vi "Table-Sort by numerical strings order.vi"(8 "error in (no error)":errorcluster, 9 "Sort By in":enum16{"row", "column"}(ring)=enum."column", 10 "Order (ascending)":enum16{"ascending", "descending"}(ring), 11 "Numerical strings table in":string[][](array[string])=[["55", "111", ""], ["3", "23", ""], ["1", "45", "123"], ["", "", ""], ["", "", ""], ["34", "", ""], ["", "", ""], ["", "", ""]]) -> (0 "error out":errorcluster, 3 "Sorted numerical strings table":string[][](array[string]))   [LabVIEW 2020]
uses:
  <userlib>/_OpenG.lib/array/array.llb/Search 1D Array (String)__ogtk.vi
  <userlib>/_OpenG.lib/array/array.llb/Delete Elements from 1D Array (String)__ogtk.vi
  <userlib>/_OpenG.lib/array/array.llb/Sort 1D Array (I32)__ogtk.vi
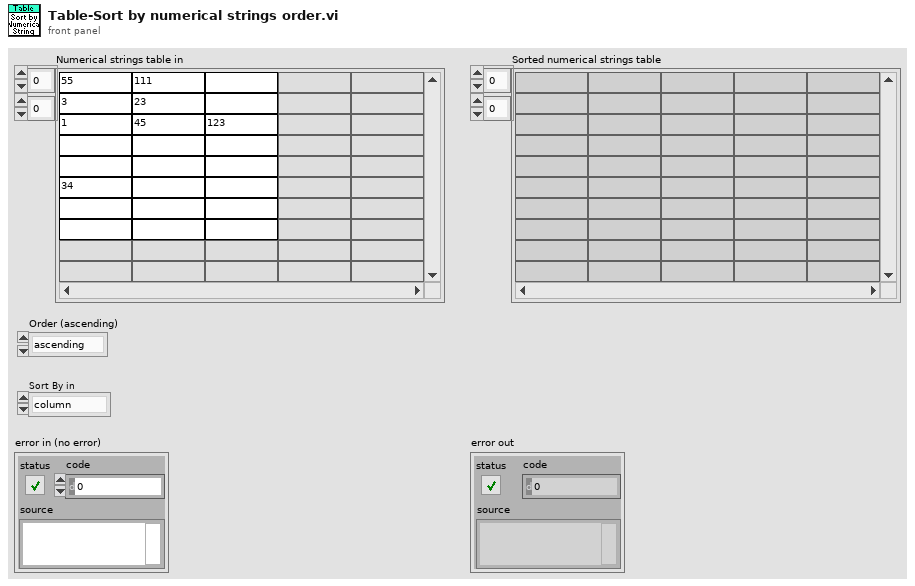
[diagram p1: front panel]
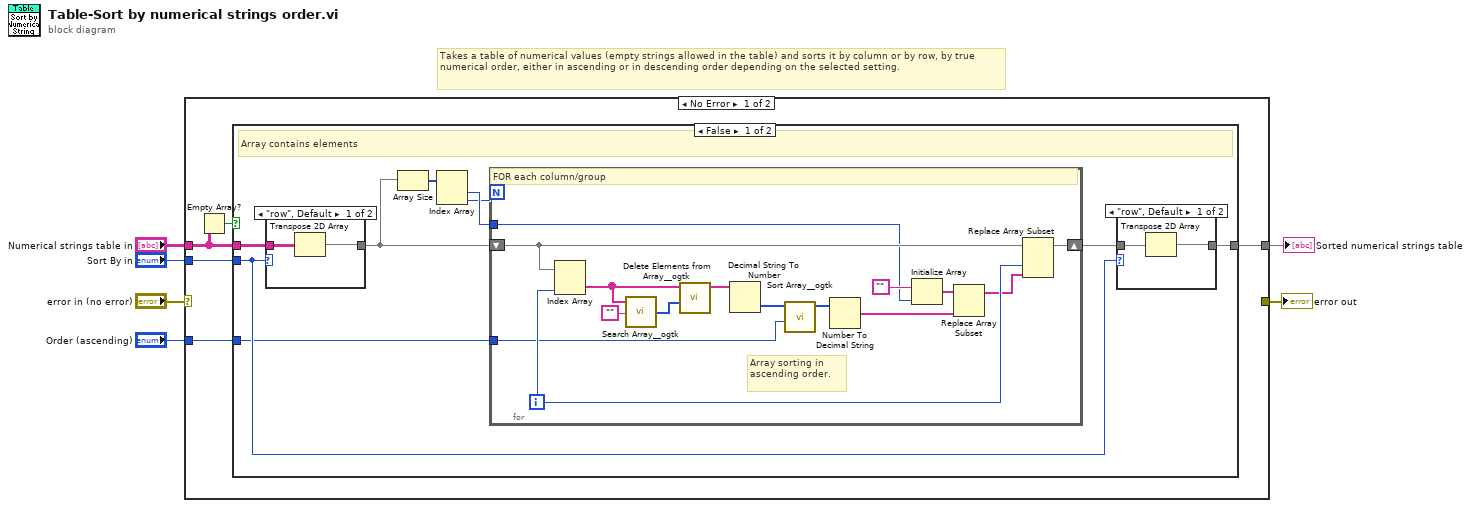
[diagram p0: block diagram]
diagram:
  # "Takes a table of numerical values (empty strings allowed in the table) and sorts it by column or by row, by true numerical order, either in ascending or in descending order depending on the selected setting."
  n1 = case shown="No Error" "error in (no error)" {
    selector: "error in (no error)" -> [_ w42]
    tunnel: [w11 _] -> w6
    tunnel: "Sort By in" -> [w10 _]
    tunnel: "Numerical strings table in" -> [w7 _]
    tunnel: "Order (ascending)" -> [w9 _]
    tunnel: [_ w42] -> w1
    frame No Error {
      n2 = Empty Array?(array=w7) -> (empty?=w8:bool)
      n3 = case shown="False" w8 {
        tunnel: [w15 _] -> w11
        tunnel: w10 -> [w14 _]
        tunnel: w7 -> [w13 _]
        tunnel: w9 -> [w12 _]
        frame False {
          # "Array contains elements"
          n4 = case shown="\"row\", Default" w14 {
            tunnel: w13 -> [w25 w26]
            tunnel: [w24 w26] -> w17
            frame "row", Default {
              n5 = Transpose 2D Array(2D array=w25) -> (transposed array=w24:string[][])
            }
            frame "column" {
            }
          }
          n6 = Array Size(array=w17) -> (size(s)=w20:i32[])
          n7 = Index Array(array=w20) -> (element #1=w19:i32, element #2=w18:i32)  [unwired: 2 in]
          n8 = for {
            N: w18 -> [_]
            shift-right: [w35] -> w16
            shift-left: w17 -> [w33]
            tunnel: w19 -> [w28]
            tunnel: w12 -> [w27]
            i -> [w34]
            # "Array sorting in ascending order."
            # "FOR each column/group"
            n9 = Index Array(array=w33, index (col)=w34) -> (element=w39:string[])  [unwired: 1 in]
            n10 = call-poly <userlib>:"Search Array__ogtk.vi"("Array"=w39, "Element Data"="") -> ("Indices of Elements"=w41:i32[])  [unwired: 7 in]
            n11 = call-poly <userlib>:"Delete Elements from Array__ogtk.vi"("indices"=w41, "array"=w39) -> ("array w/ subset deleted"=w38:string[])  [unwired: 8 in, 1 out]
            n12 = Decimal String To Number(string=w38) -> (number=w37:i32[])  [unwired: 2 in, 1 out]
            n13 = call-poly <userlib>:"Sort Array__ogtk.vi"("Order"=w27, "Array in"=w37) -> ("Sorted Array out"=w36:i32[])  [unwired: 8 in, 1 out]
            n14 = Number To Decimal String(number=w36) -> (decimal integer string=w30:string[])  [unwired: 1 in]
            n15 = Initialize Array("", w28) -> (w31:string[])
            n16 = Replace Array Subset(array=w31, new element=w30) -> (w29:string[])  [unwired: 1 in]
            n17 = Replace Array Subset(array=w33, new element=w29, index (col)=w34) -> (w35:string[][])  [unwired: 1 in]
          }
          n18 = case shown="\"row\", Default" w14 {
            tunnel: w16 -> [w22 w23]
            tunnel: [w21 w23] -> w15
            frame "row", Default {
              n19 = Transpose 2D Array(2D array=w22) -> (transposed array=w21:string[][])
            }
            frame "column" {
            }
          }
        }
        frame True {
          # "Array is empty"
        }
      }
    }
    frame Error {
    }
  }
  "Sorted numerical strings table" <- w6
  "error out" <- w1
